vi "Search 1D Array Partial Match.vi"(5 "Ignore case? (F)":bool, 7 "Method (Contains Search String)":T1(ring), 10 "Item to Search":string, 11 "Search Strings":string[](array[string])) -> (3 "First Index Found":i32)   [LabVIEW 2017, in "Front Panel Publisher.lvlib"]
doc: "This VI will search a 1D array of sting<B>Search Strings</B> using <B>Item to Search</B>. This search will be performed attempting to find the first item in <B>Search Strings</B> that contains the same text as some of the text in <B>Item to Search</B>. In this way <B>Item to Search</B> can be a much longer string than <B>Search Strings</B>. This array will be searched using the method defined in <b>Method</b>. The output of <B>First Index Found</B> will contain the index of <B>Search Strings</B> that first met the search criteria.\n\nThis VI can search for the element that contains the search string, start with the search string, or end with the search string.\n\nThe search can also be modified to <b>Ignore case</b> which will cause the search string to ignore capitialization."
uses:
  Front Panel Publisher.lvlib
  <userlib>/_OpenG.lib/array/array.llb/Search 1D Array (Boolean)__ogtk.vi
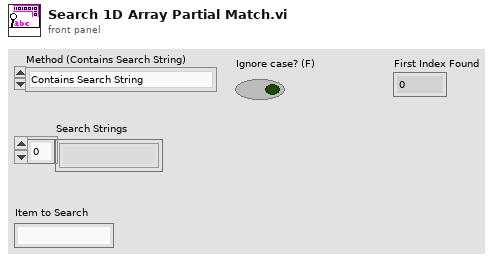
[diagram p1: front panel]
types:
  T1 = enum16{"Contains Search String", "Starts With Search String", "Ends With Search String"}
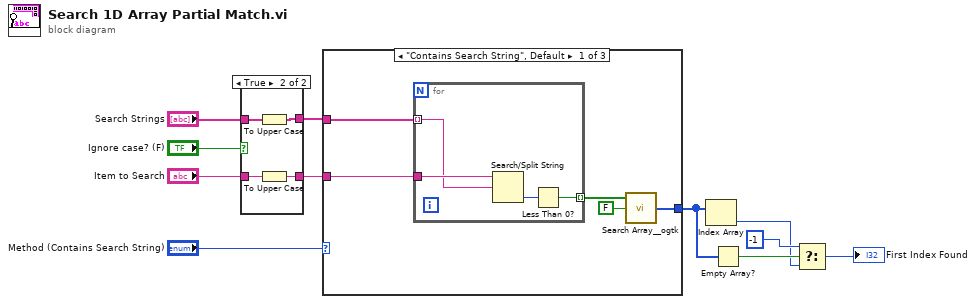
[diagram p0: block diagram]
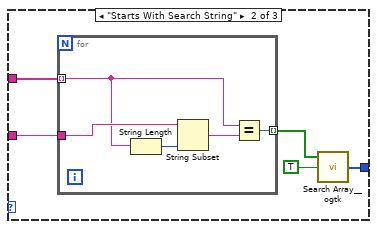
[diagram p3: hidden frame]
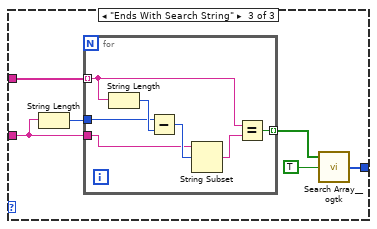
[diagram p4: hidden frame]
diagram:
  n1 = case shown="True" "Ignore case? (F)" {
    tunnel: "Item to Search" -> [w12 w15]
    tunnel: "Search Strings" -> [w13 w17]
    tunnel: [w13 w16] -> w8
    tunnel: [w12 w14] -> w7
    frame False {
    }
    frame True {
      n2 = To Upper Case(1:w17) -> (0:w16:string[])
      n3 = To Upper Case(1:w15) -> (0:w14:string)
    }
  }
  n4 = case shown="\"Contains Search String\", Default" "Method (Contains Search String)" {
    tunnel: w7 -> [w22 w30 w41]
    tunnel: w8 -> [w21 w31 w42]
    tunnel: [w18 w27 w37] -> w5
    frame "Contains Search String", Default {
      n5 = for {
        tunnel: w21 -> [w23] mode=indexing
        tunnel: w22 -> [w24]
        tunnel: [w25] -> w20 mode=indexing
        n6 = Search/Split String(string=w24, search string/char (-)=w23) -> (offset of match=w26:i32)  [unwired: 1 in, 2 out]
        n7 = Less Than 0?(x=w26) -> (x < 0?=w25:bool)
      }
      n8 = call-poly <userlib>:"Search Array__ogtk.vi"("Array"=w20, "Element Data"=FALSE) -> ("Indices of Elements"=w18:i32[])  [unwired: 7 in]
    }
    frame "Starts With Search String" {
      n9 = for {
        tunnel: w31 -> [w32] mode=indexing
        tunnel: w30 -> [w35]
        tunnel: [w36] -> w29 mode=indexing
        n10 = String Length(string=w32) -> (length=w33:i32)
        n11 = String Subset(string=w35, length (rest)=w33) -> (substring=w34:string)  [unwired: 1 in]
        n12 = Equal?(x=w32, y=w34) -> (x = y?=w36:bool)
      }
      n13 = call-poly <userlib>:"Search Array__ogtk.vi"("Array"=w29, "Element Data"=TRUE) -> ("Indices of Elements"=w27:i32[])  [unwired: 7 in]
    }
    frame "Ends With Search String" {
      n14 = String Length(string=w41) -> (length=w40:i32)
      n15 = for {
        tunnel: w42 -> [w45] mode=indexing
        tunnel: w41 -> [w44]
        tunnel: [w49] -> w38 mode=indexing
        tunnel: w40 -> [w46]
        n16 = String Length(string=w45) -> (length=w47:i32)
        n17 = Subtract(x=w46, y=w47) -> (x-y=w48:i32)
        n18 = String Subset(string=w44, offset (0)=w48) -> (substring=w43:string)  [unwired: 1 in]
        n19 = Equal?(x=w45, y=w43) -> (x = y?=w49:bool)
      }
      n20 = call-poly <userlib>:"Search Array__ogtk.vi"("Array"=w38, "Element Data"=TRUE) -> ("Indices of Elements"=w37:i32[])  [unwired: 7 in]
    }
  }
  n21 = Index Array(array=w5) -> (element=w2:i32)  [unwired: 1 in]
  n22 = Empty Array?(array=w5) -> (empty?=w4:bool)
  n23 = Select(t=-1, s=w4, f=w2) -> (s? t:f=→"First Index Found":i32)
